vi "MapCompare.vi"(4 "Scan Period":dbl format="%.2f", 5 "Previous Scan Value":dbl format="%.2f", 6 "Present scan array":dbl[](array[numeric]) format="%.2f", 7 "Value to Output":dbl format="%.2f", 8 "Ch Description":T1={"Ch Name"="Vib:NDE:MapCheck", "Type"="Run VI Named:", "Function"=enum."Analogue Input", "Ch State"=enum."On", "Calibration type"="Raw", "A"=0.15, "B"=10.0, "C"=0.0, "D"=0.0, "Comments"="MapCompare.vi", "Address"={"Main"=0, "Ch."=0, "Sub"=0, "Port Name"=""}, "String"="vibMapEastNDE.xls;VFD-E:Measured:RPM;VFD-E:Vibro:NDE(RMSmm/s)", "Duty"=65535} {"Duty" format="%016b"; "D" format="%#_5g"; "C" format="%#_5g"; "B" format="%#_5g"; "A" format="%#_5g"}, 9 "Ch names":string[](array[string])) -> (0 "Scan comment":string, 1 "Output":dbl format="%.3f", 3 "HelpText":string="Compares values retrieved from earlier channel with \"map\" of historic values, and warns if new values are out of spec.\nThis help text needs to be made dynamic.\nAcceptable radius (in Y axis units) is in A, minimum number of historic points is in B.")   [LabVIEW 2022 SP3]
uses:
  ADAM Client/Sub VIs/ADAM Controls/Ch_description_ADAM.ctl
  ADAM Client/Sub VIs/ADAM Controls/Module_type_ADAM.ctl
  ADAM Client/Sub VIs/ADAM Controls/Function_ADAM.ctl
  ADAM Client/Sub VIs/ADAM Controls/Channel_State.ctl
  ADAM Client/Sub VIs/ADAM Controls/Calib_type_ADAM.ctl
  ADAM Client/Sub VIs/ADAM Controls/Address.ctl
  ADAM Client/Sub VIs/ADAM Controls/Search_mode.ctl
  08b3dcb4-80c0-6749-b1ed-dba7bf5e912d.vi
  Anemometry/Anemometry Sub Vis/Globals/Constants_global.vi
  <vilib>/Utility/file.llb/Read Delimited Spreadsheet (DBL).vi
  <vilib>/Comparison/Less/Less Functor/Less Functor.lvclass
  <vilib>/Analysis/NI_AALBase.lvlib
panel:
  in  "forceReload":bool
  in  "forcePlot":bool
  out "warn":bool
  out "BpointsMaxRadius":dbl
  out "x/y":dbl
  out "BpointsMedianRadius":dbl format="%0.2f"
  out "nPointsInsideA":dbl
  out "Yval":dbl
  out "Xval":dbl
  out "Ych":string
  out "Xch":string
  out "mapName":string
  out "XY Graph":cluster{"all rows":dbl[], "all rows":dbl[]}[](graph)
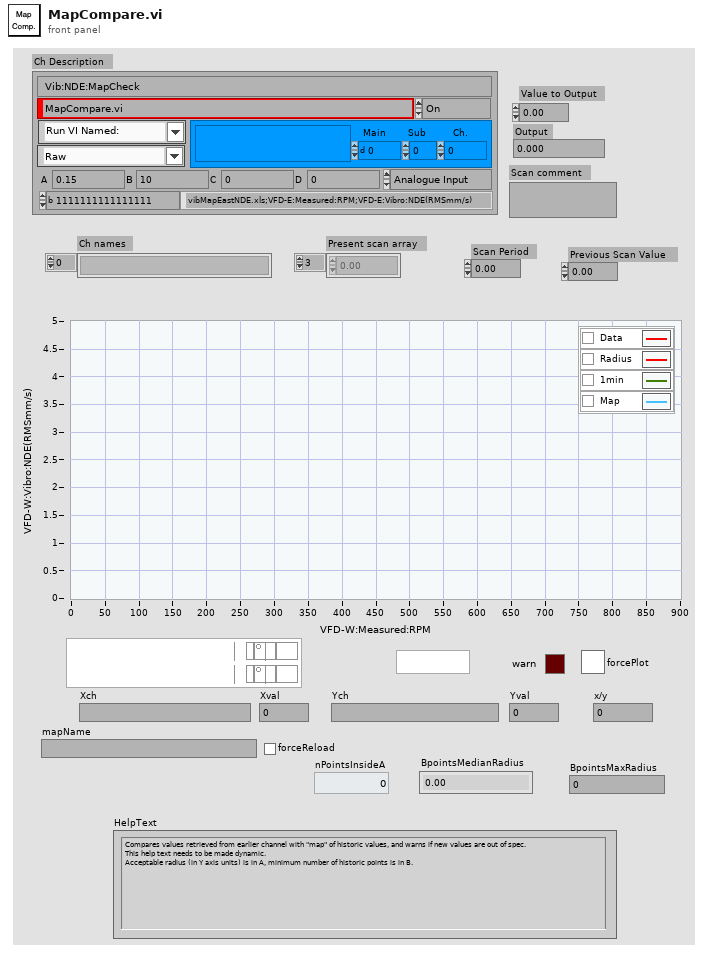
[diagram p1: front panel]
types:
  T1 = typedef "Ch_description_ADAM.ctl" = cluster{"Ch Name":string, "Type":T2, "Function":T3, "Ch State":T4, "Calibration type":T5, "A":dbl, "B":dbl, "C":dbl, "D":dbl, "Comments":string, "Address":T6, "String":string, "Duty":u16}
  T2 = typedef "Module_type_ADAM.ctl" = string
  T3 = typedef "Function_ADAM.ctl" = enum16{"Analogue Input", "Digital Input", "Event counter", "Event rate", "Analogue Output", "Digital Output", "Relay Output"}
  T4 = typedef "Channel_State.ctl" = enum16{"On", "Off", "Always On", "Always Off"}
  T5 = typedef "Calib_type_ADAM.ctl" = string
  T6 = typedef "Address.ctl" = cluster{"Main":i32, "Ch.":i32, "Sub":i32, "Port Name":string}
  T7 = typedef "Search_mode.ctl" = enum16{"Between times", "All Times"}
  T8 = cluster{"Output array":dbl[], "Output array":dbl[]}
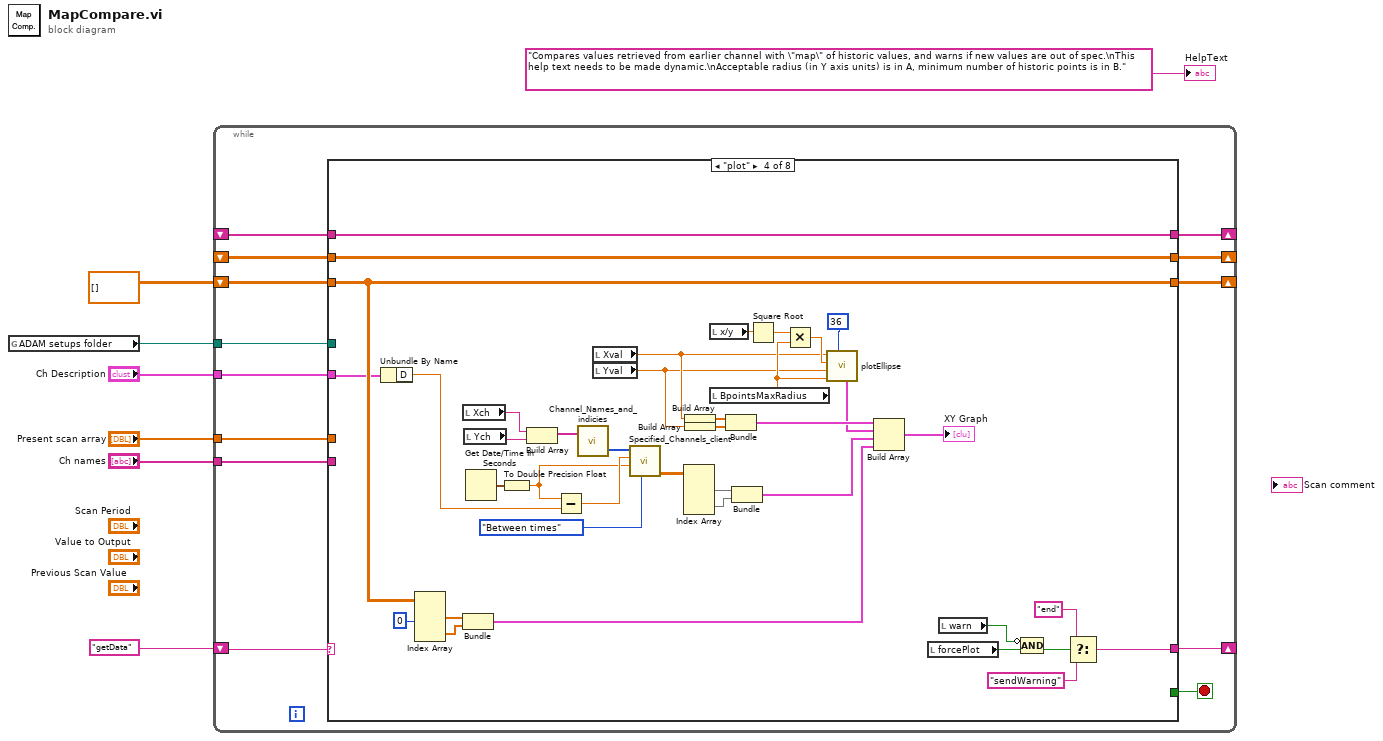
[diagram p0: block diagram]
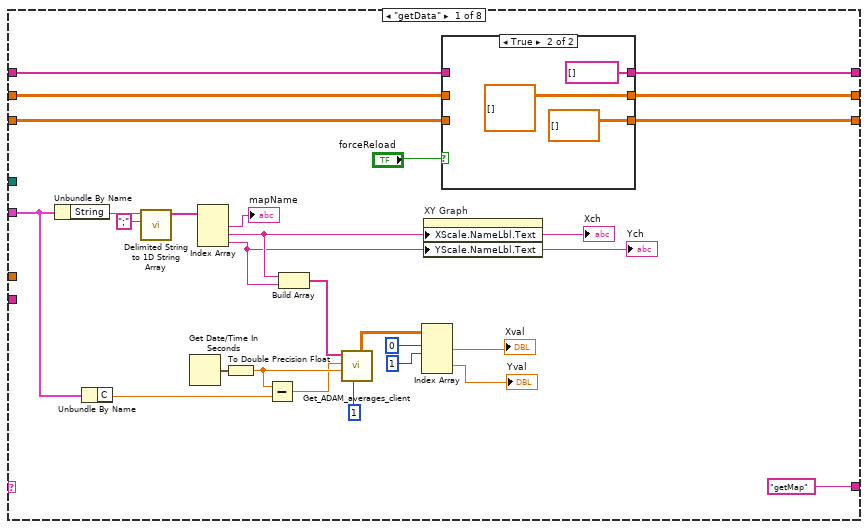
[diagram p2: hidden frame]
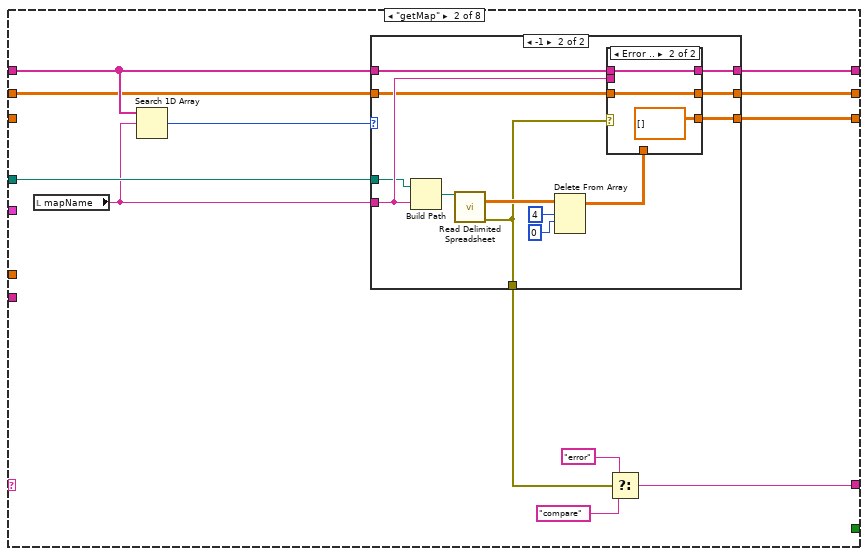
[diagram p4: hidden frame]
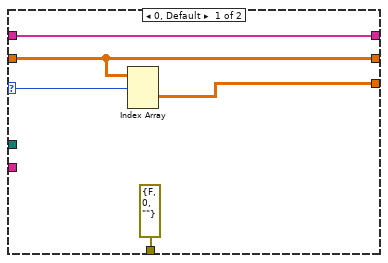
[diagram p5: hidden frame]
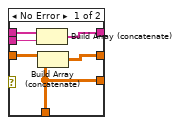
[diagram p6: hidden frame]
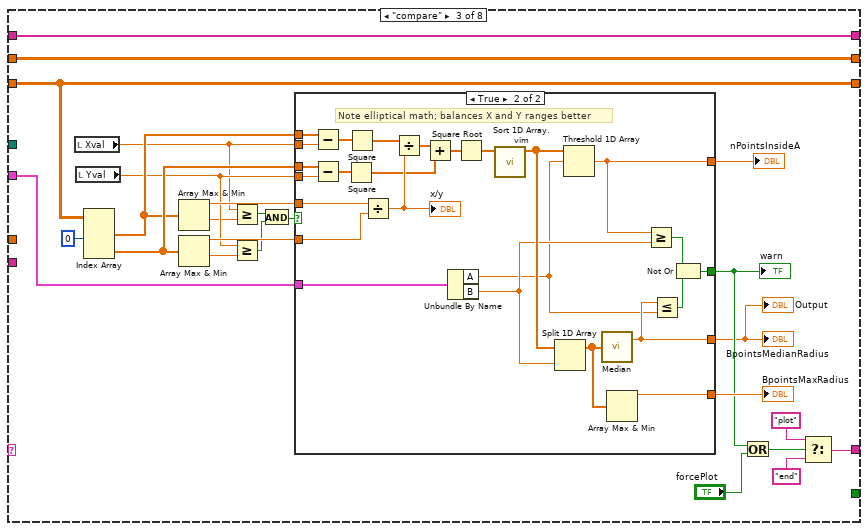
[diagram p7: hidden frame]
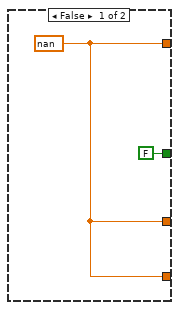
[diagram p8: hidden frame]
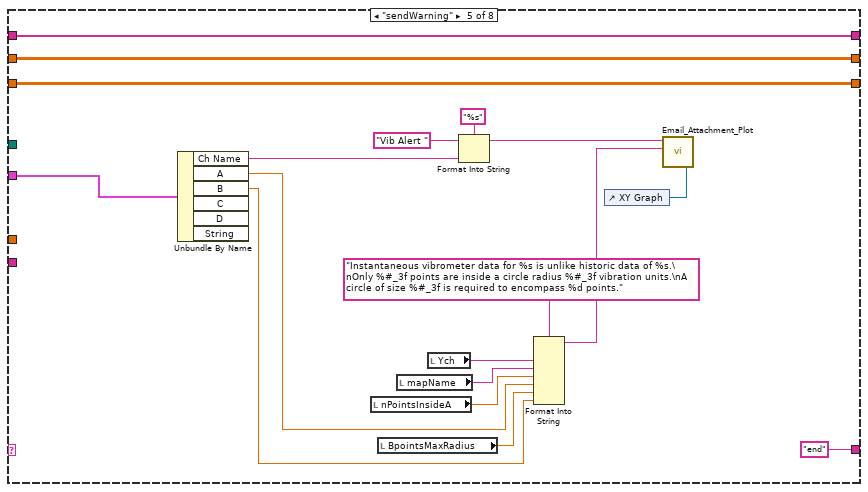
[diagram p9: hidden frame]
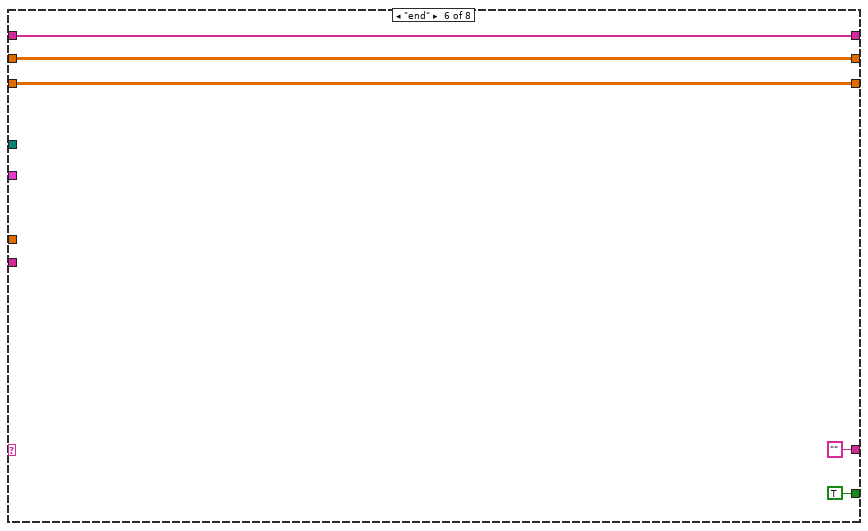
[diagram p10: hidden frame]
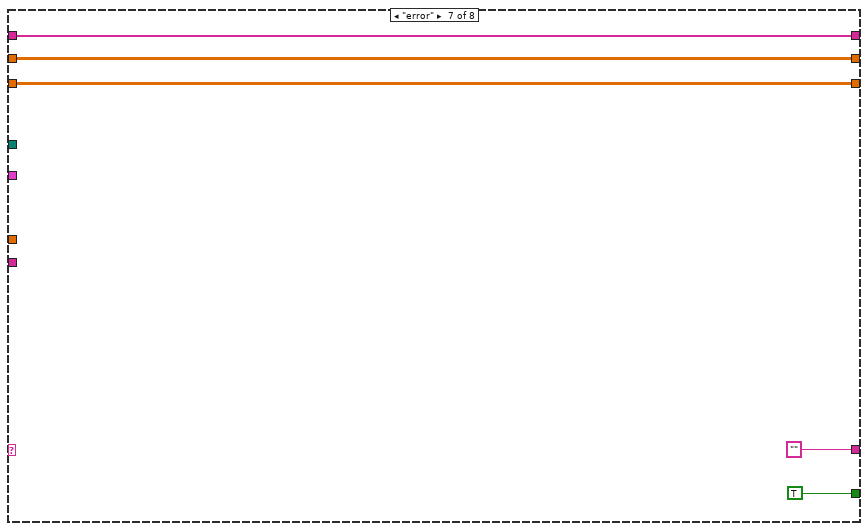
[diagram p11: hidden frame]
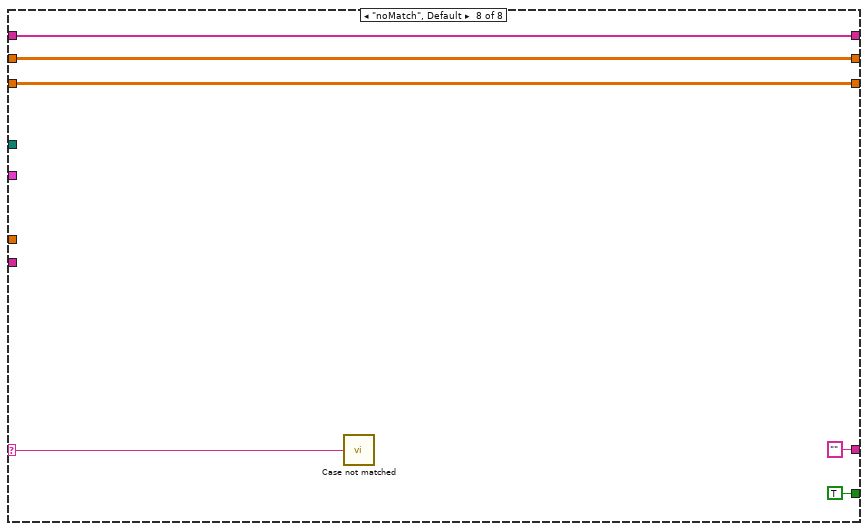
[diagram p12: hidden frame]
diagram:
  n1 = global read "Constants_global.vi" "ADAM setups folder"() -> (w4:path)
  n2 = while {
    shift-right: [w10] -> _
    shift-left: "getData" -> [w20]
    tunnel: "Ch Description" -> [w18]
    shift-right: [w16] -> _
    shift-left: _ -> [w17]
    shift-right: [w14] -> _
    shift-left: _ -> [w15]
    shift-right: [w13] -> _
    shift-left: dbl[][] [] ("all rows") -> [w12]
    tunnel: w4 -> [w11]
    tunnel: "Ch names" -> [w9]
    tunnel: "Present scan array" -> [w8]
    stop <- w19 stop-if-true
    n3 = case shown="\"plot\"" w20 {
      selector: w20 -> [_ _ _ _ _ _ _ w211]
      tunnel: [_ _ _ _ _ TRUE TRUE TRUE] -> w19
      tunnel: w18 -> [w30 _ w108 w149 w195 _ _ _]
      tunnel: w17 -> [w39 w63 w116 w182 w200 w205 w210 w216]
      tunnel: [w40 w62 w116 w182 w200 w205 w210 w216] -> w16
      tunnel: w15 -> [w37 w61 w115 w181 w199 w204 w209 w215]
      tunnel: [w38 w60 w115 w181 w199 w204 w209 w215] -> w14
      tunnel: [w36 w59 w110 w177 w198 w203 w208 w214] -> w13
      tunnel: w12 -> [w35 _ w110 w177 w198 w203 w208 w214]
      tunnel: w11 -> [_ w58 _ _ _ _ _ _]
      tunnel: ["getMap" w56 w98 w151 "end" "" ("f") "" "" ("f")] -> w10
      tunnel: w9 -> [_ _ _ _ _ _ _ _]
      tunnel: w8 -> [_ _ _ _ _ _ _ _]
      frame "getData" {
        n4 = Unbundle By Name(w30) -> ("String"=w46:string)
        n5 = Unbundle By Name(w30) -> ("C"=w28:dbl)
        n6 = call <vilib>:"Delimited String to 1D String Array.vi"("delimiter"=";", "delimited string"=w46) -> ("string array"=w42:string[])  [unwired: 9 in]
        n7 = Get Date/Time In Seconds() -> (seconds since 1Jan1904=w32:timestamp)
        n8 = Index Array(array=w42) -> (element #1=→"mapName":string, element #2=w22:string, element #3=w21:string)  [unwired: 3 in]
        "Xch" <- w22
        "Ych" <- w21
        n9 = To Double Precision Float(number=w32) -> (double precision float=w29:dbl)
        n10 = Subtract(x=w29, y=w28) -> (x-y=w27:dbl)
        n11 = Build Array(w22, w21) -> (w33:string[])
        n12 = call "Get_ADAM_averages_client.vi"("No of averages"=1, "End time"=w29, "Start time"=w27, "ADAM Ch Names"=w33) -> ("DBL values"=w34:dbl[][])  [unwired: 3 in, 4 out]
        n13 = Index Array(array=w34, index (row) #1=0 ("disabled index (row)"), index (col) #1=1 ("disabled index (col)")) -> (element #1=→"Xval":dbl, element #2=→"Yval":dbl)  [unwired: 2 in]
        n14 = property on="XY Graph" class="XYGraph (strict)"("XScale.NameLbl.Text"=w22, "YScale.NameLbl.Text"=w21) -> ()  [unwired: 2 in, 2 out]
        n15 = case shown="True" "forceReload" {
          tunnel: [w49 string[] []] -> w40
          tunnel: w39 -> [w49 _]
          tunnel: [w48 dbl[][][] []] -> w38
          tunnel: w37 -> [w48 _]
          tunnel: [w47 dbl[][] [] ("all rows")] -> w36
          tunnel: w35 -> [w47 _]
          frame False {
          }
          frame True {
          }
        }
      }
      frame "getMap" {
        n16 = local read "mapName"() -> (w53:string)
        n17 = Search 1D Array(1D array=w63, element=w53) -> (index of element=w64:i32)  [unwired: 1 in]
        n18 = case shown="-1" w64 {
          selector: w64 -> [w69 _]
          tunnel: w53 -> [_ w77]
          tunnel: w63 -> [w66 w78]
          tunnel: [w66 w76] -> w62
          tunnel: w61 -> [w67 w75]
          tunnel: [w67 w74] -> w60
          tunnel: [w68 w70] -> w59
          tunnel: w58 -> [_ w72]
          tunnel: [errorcluster {"status"=FALSE, "code"=0, "source"=""} ("error out") w71] -> w57
          frame 0, Default {
            n19 = Index Array(array=w67, index (dim 0)=w69) -> (element=w68:dbl[][])  [unwired: 2 in]
          }
          frame -1 {
            n20 = Build Path(base path=w72, name or relative path=w77) -> (appended path=w79:path)
            n21 = call-poly <vilib>:"Read Delimited Spreadsheet.vi"("file path (dialog if empty)"=w79) -> ("all rows"=w80:dbl[][], "error out"=w71:errorcluster)  [unwired: 9 in, 4 out]
            n22 = Delete From Array(array=w80, length=4, index (row)=0) -> (array with subset deleted=w73:dbl[][])  [unwired: 1 in, 1 out]
            n23 = case shown="Error .." w71 {
              tunnel: w78 -> [w88 w91]
              tunnel: w77 -> [w87 _]
              tunnel: [w86 w91] -> w76
              tunnel: w75 -> [w85 w90]
              tunnel: [w84 w90] -> w74
              tunnel: w73 -> [w83 _]
              tunnel: [w83 dbl[][] [] ("all rows")] -> w70
              frame No Error {
                n24 = Build Array (concatenate)(w88, w87) -> (w86:string[])
                n25 = Build Array (concatenate)(w85, w83) -> (w84:dbl[][][])
              }
              frame Error {
              }
            }
          }
        }
        n26 = Select(t="error", s=w57, f="compare") -> (s? t:f=w56:string)
      }
      frame "compare" {
        n27 = local read "Xval"() -> (w103:dbl)
        n28 = local read "Yval"() -> (w105:dbl)
        n29 = Index Array(array=w110, index (col) #1=0 ("disabled index (col)")) -> (element #1=w109:dbl[], element #2=w112:dbl[])  [unwired: 3 in]
        n30 = Array Max & Min(array=w109) -> (max value=w113:dbl, min value=w102:dbl)  [unwired: 2 out]
        n31 = Array Max & Min(array=w112) -> (max value=w114:dbl, min value=w104:dbl)  [unwired: 2 out]
        n32 = Greater Or Equal?(x=w103, y=w102) -> (x >= y?=w101:bool)
        n33 = Greater Or Equal?(x=w105, y=w104) -> (x >= y?=w99:bool)
        n34 = And(x=w101, y=w99) -> (x .and. y?=w100:bool)
        n35 = case shown="True" w100 {
          tunnel: w114 -> [_ w139]
          tunnel: w113 -> [_ w138]
          tunnel: w112 -> [_ w137]
          tunnel: w103 -> [_ w136]
          tunnel: w109 -> [_ w135]
          tunnel: w105 -> [_ w134]
          tunnel: w108 -> [_ w128]
          tunnel: [w118 w126] -> w107
          tunnel: [w118 w125] -> w106
          tunnel: [w118 w124] -> w94
          tunnel: [FALSE w119] -> w96
          frame False {
            w118 = nan
          }
          frame True {
            # "Note elliptical math; balances X and Y ranges better"
            n36 = Subtract(x=w135, y=w136) -> (x-y=w132:dbl[])
            n37 = Subtract(x=w137, y=w134) -> (x-y=w140:dbl[])
            n38 = Square(x=w140) -> (x^2=w141:dbl[])
            n39 = Square(x=w132) -> (x^2=w131:dbl[])
            n40 = Divide(x=w138, y=w139) -> (x/y=w143:dbl)
            "x/y" <- w143
            n41 = Divide(x=w131, y=w143) -> (x/y=w130:dbl[])
            n42 = Add(x=w130, y=w141) -> (x+y=w142:dbl[])
            n43 = Unbundle By Name(w128) -> ("A"=w122:dbl, "B"=w123:dbl)
            n44 = Square Root(x=w142) -> (sqrt(x)=w133:dbl[])
            n45 = call "Sort 1D Array.vim"("unsorted array"=w133) -> ("sorted array"=w129:dbl[])  [unwired: 10 in]
            n46 = Split 1D Array(array=w129, index=w123) -> (first subarray=w127:dbl[])  [unwired: 1 out]
            n47 = Threshold 1D Array(2:w122, 3:w129) -> (0:w125:dbl)  [unwired: 1 in]
            n48 = call <vilib>:"Median.vi"("X"=w127) -> ("median"=w124:dbl)  [unwired: 1 out]
            n49 = Array Max & Min(array=w127) -> (max value=w126:dbl)  [unwired: 3 out]
            n50 = Greater Or Equal?(x=w125, y=w123) -> (x >= y?=w121:bool)
            n51 = Less Or Equal?(x=w124, y=w122) -> (x <= y?=w120:bool)
            n52 = Not Or(1:w120, 2:w121) -> (0:w119:bool)
          }
        }
        "nPointsInsideA" <- w106
        "BpointsMedianRadius" <- w94
        "BpointsMaxRadius" <- w107
        "warn" <- w96
        "Output" <- w94
        n53 = Or(x=w96, y="forcePlot") -> (x .or. y?=w93:bool)
        n54 = Select(t="plot", s=w93, f="end") -> (s? t:f=w98:string)
      }
      frame "plot" {
        n55 = Unbundle By Name(w149) -> ("D"=w148:dbl)
        n56 = Index Array(array=w177, index (col) #1=0 ("disabled index (col)")) -> (element #1=w179:dbl[], element #2=w178:dbl[])  [unwired: 3 in]
        n57 = local read "Xch"() -> (w162:string)
        n58 = Bundle("all rows"=w179, "all rows"=w178) -> (w156:cluster{"all rows":dbl[], "all rows":dbl[]})  [unwired: 1 in]
        n59 = local read "Ych"() -> (w161:string)
        n60 = Get Date/Time In Seconds() -> (seconds since 1Jan1904=w164:timestamp)
        n61 = To Double Precision Float(number=w164) -> (double precision float=w147:dbl)
        n62 = Build Array(w162, w161) -> (w146:string[])
        n63 = Subtract(x=w147, y=w148) -> (x-y=w163:dbl)
        n64 = call "Channel_Names_and_indicies.vi"("Desired Ch Names"=w146) -> ("Indicies"=w145:i32[])  [unwired: 1 in, 1 out]
        n65 = local read "Xval"() -> (w167:dbl)
        n66 = local read "Yval"() -> (w166:dbl)
        n67 = call "Specified_Channels_client.vi"("Mode"=Search_mode."Between times", "End time"=w147, "Start time"=w163, "ADAM Index array"=w145) -> ("Output array"=w158:dbl[][])  [unwired: 3 in, 4 out]
        n68 = Index Array(array=w158) -> (element #1=w159:dbl[], element #2=w160:dbl[])  [unwired: 4 in]
        n69 = Build Array(w167) -> (w168:dbl[])
        n70 = Build Array(w166) -> (w165:dbl[])
        n71 = local read "x/y"() -> (w174:dbl)
        n72 = local read "BpointsMaxRadius"() -> (w171:dbl)
        n73 = Bundle(w168, w165) -> (w175:cluster{dbl[], dbl[]})  [unwired: 1 in]
        n74 = Bundle("Output array"=w159, "Output array"=w160) -> (w157:T8)  [unwired: 1 in]
        n75 = Square Root(x=w174) -> (sqrt(x)=w170:dbl)
        n76 = Multiply(x=w170, y=w171) -> (x*y=w169:dbl)
        n77 = call "plotEllipse.vi"("nPoints"=36, "Yradius"=w171, "Ycentre"=w166, "Xradius"=w169, "Xcentre"=w167) -> ("plottable"=w172:cluster{"Array":dbl[], "Array":dbl[]})  [unwired: 4 in, 2 out]
        n78 = Build Array(w175, w172, w157, w156) -> (→"XY Graph":cluster{"all rows":dbl[], "all rows":dbl[]}[])
        n79 = local read "forcePlot"() -> (w155:bool)
        n80 = local read "warn"() -> (w153:bool)
        n81 = Compound Arithmetic op=AND(invert w153, w155) -> (w154:bool)
        n82 = Select(t="end", s=w154, f="sendWarning") -> (s? t:f=w151:string)
      }
      frame "sendWarning" {
        n83 = Unbundle By Name(w195) -> ("Ch Name"=w192:string, "A"=w185:dbl, "B"=w183:dbl)  [unwired: 3 out]
        n84 = local read "nPointsInsideA"() -> (w186:dbl)
        n85 = local read "BpointsMaxRadius"() -> (w184:dbl)
        n86 = local read "mapName"() -> (w187:string)
        n87 = local read "Ych"() -> (w190:string)
        n88 = Format Into String(format string="%s", initial string="Vib Alert " ("subject"), w192) -> (resulting string=w193:string)  [unwired: 1 in, 1 out]
        n89 = Format Into String(format string="Instantaneous vibrometer data for %s is unlike historic data of %s.\nOnly %#_3f points are inside a circle radius %#_3f vibration units.\nA circle of size %#_3f is required to encompass %d points.", w190, w187, w186, w185, w184, w183) -> (resulting string=w191:string)  [unwired: 2 in, 1 out]
        n90 = control-ref of="XY Graph"() -> (w196:refnum<vi>)
        n91 = call "Email_Attachment_Plot.vi"("controlRef"=w196, "message"=w191, "subject"=w193) -> ()  [unwired: 4 in]
      }
      frame "end" {
      }
      frame "error" {
      }
      frame "noMatch", Default {
        n92 = call "Case not matched.vi"("Case Name not Matched"=w211) -> ()
      }
    }
  }
  "HelpText" <- "Compares values retrieved from earlier channel with \"map\" of historic values, and warns if new values are out of spec.\nThis help text needs to be made dynamic.\nAcceptable radius (in Y axis units) is in A, minimum number of historic points is in B." ("HelpText")
